vi "Save Formula Aliases.vi"(0 "Dialog? (F)":bool, 5 "Aliases Array":string[](array[string]), 7 "Definitions Array":string[](array[string]), 9 "Descriptions Array":string[](array[string]), 11 "error in (no error)":errorcluster) -> (4 "File Content":string[](array[string]), 15 "error out":errorcluster)   [LabVIEW 2021, in "Formula.lvlib"]
uses:
  Formula.lvlib
  Files/Files.lvlib
  Error/Error.lvlib
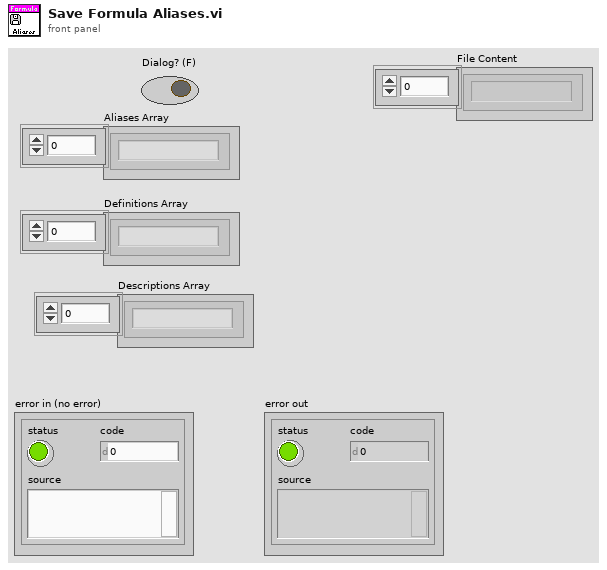
[diagram p1: front panel]
types:
  T1 = enum16{"open", "replace", "create", "open or create", "replace or create", "replace or create with confirmation"}
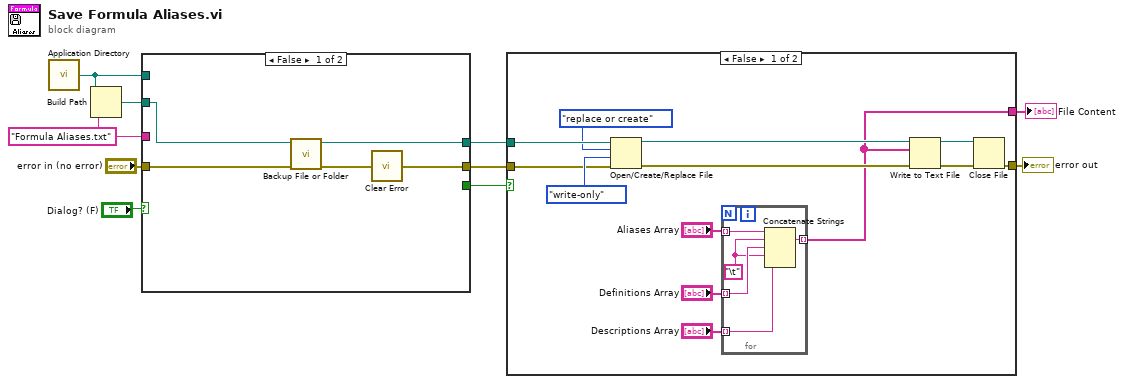
[diagram p0: block diagram]
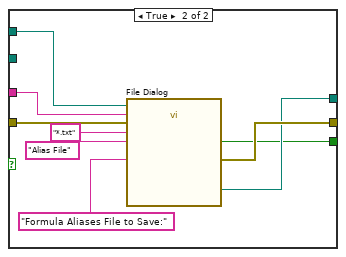
[diagram p3: hidden frame]
diagram:
  w6 = "Formula Aliases.txt" ("name or relative path")
  n1 = call <vilib>:"Application Directory.vi"() -> ("Application Directory"=w7:path)
  n2 = Build Path(base path=w7, name or relative path=w6) -> (appended path=w5:path)
  n3 = case shown="False" "Dialog? (F)" {
    tunnel: "error in (no error)" -> [w15 w24]
    tunnel: w7 -> [_ w20]
    tunnel: w6 -> [_ w19]
    tunnel: w5 -> [w14 _]
    tunnel: [w11 w18] -> w3
    tunnel: [w13 w17] -> w4
    tunnel: [_ w16] -> w2
    frame False {
      n4 = call "Backup File or Folder.vi"("error in (no error)"=w15, "File/Directory Path"=w14) -> ("error out"=w12:errorcluster, "File/Directory Path (dup)"=w13:path)  [unwired: 8 in]
      n5 = call "Clear Error.vi"("Error In"=w12) -> ("no Error Out"=w11:errorcluster)  [unwired: 8 in]
    }
    frame True {
      n6 = call "File Dialog"("start path"=w20, "prompt"="Formula Aliases File to Save:", "default name"=w19, "error in"=w24, "pattern (all files)"="*.txt", "pattern label"="Alias File") -> ("selected path"=w17:path, "cancelled"=w16:bool, "error out"=w18:errorcluster)  [unwired: 6 in, 1 out]
    }
  }
  n7 = case shown="False" w2 {
    tunnel: [w36 w43] -> w10
    tunnel: w4 -> [w31 _]
    tunnel: w3 -> [w28 w43]
    tunnel: [w25 _] -> w1
    frame False {
      n8 = Open/Create/Replace File(file path (use dialog)=w31, error in=w28, operation (0:open)=T1."replace or create", access (0:read/write)=enum16{"read/write", "read-only", "write-only"}."write-only") -> (refnum out=w26:refnum<file>, error out=w27:errorcluster)  [unwired: 2 in, 1 out]
      n9 = for {
        tunnel: "Aliases Array" -> [w42] mode=indexing
        tunnel: "Definitions Array" -> [w41] mode=indexing
        tunnel: [w40] -> w25 mode=indexing
        tunnel: "Descriptions Array" -> [w38] mode=indexing
        w39 = "\t"
        n10 = Concatenate Strings(w42, w39, w41, w39, w38) -> (w40:string)
      }
      n11 = Write to Text File(file (use dialog)=w26, text=w25, error in=w27) -> (refnum out=w34:refnum<file>, error out=w35:errorcluster)  [unwired: 1 in, 1 out]
      n12 = Close File(refnum=w34, error in=w35) -> (error out=w36:errorcluster)  [unwired: 1 out]
    }
    frame True {
    }
  }
  "error out" <- w10
  "File Content" <- w1
